vi "ConvertPB_Triggers.vi"(0 "PB VLIW Array in":T2(array[cluster]) {"Output Bits" format="%x"}, 1 "Definitions":T1={"External MemorySize"=32768, "Internal Memory Size"=512, "Overhead Ticks"=3, "Min Delay Loops"=3, "Loop Count Correction"=1, "Long Delay Loop Count Correction"=2, "Min Instruction Ticks"=6, "Long Delay Ticks"=4294967295, "Clock Period (s)"=1e-08, "Overhead Time (s)"=3e-08, "Min Instruction Cycle Time (s)"=9e-08, "Long Delay Time (s) "=42.94967298} {"Long Delay Time (s)" format="%.8p"; "Min Instruction Cycle Time (s)" format="%.0p"; "Overhead Time (s)" format="%.0p"; "Clock Period (s)" format="%.0p"; "Long Delay Ticks" format="%.0x"}, 2 "error in (no error)":errorcluster, 3 "Full trigger mask":u32 format="%x") -> (5 "PB VLIW Array out":T2(array[cluster]) {"Output Bits" format="%x"}, 6 "error out":errorcluster)   [LabVIEW 2013, in "PulseBlaster.lvlib"]
uses:
  PulseBlaster.lvlib
panel:
  in  "BeginLoop pointer":u32
  # "(Period*Long D Ticks)+Overhead time"
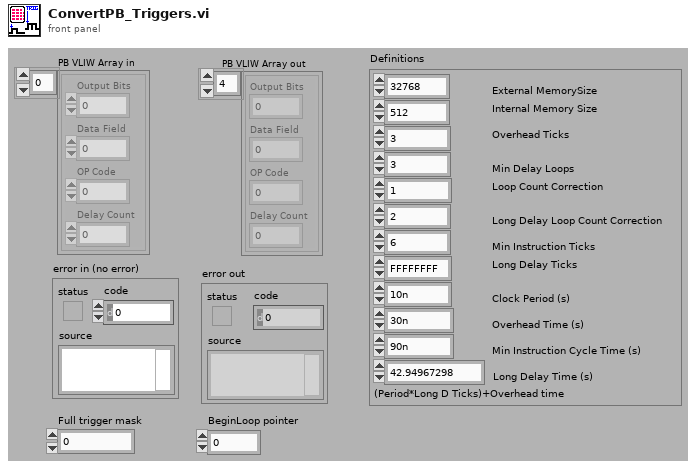
[diagram p1: front panel]
types:
  T1 = cluster{"External MemorySize":u16, "Internal Memory Size":u16, "Overhead Ticks":u8, "Min Delay Loops":u8, "Loop Count Correction":u8, "Long Delay Loop Count Correction":u8, "Min Instruction Ticks":u8, "Long Delay Ticks":u64, "Clock Period (s)":dbl, "Overhead Time (s)":dbl, "Min Instruction Cycle Time (s)":dbl, "Long Delay Time (s) ":dbl}
  T2 = cluster{"Output Bits":u32, "Data Field":u32, "OP Code":u8, "Delay Count":u64}[]
  T3 = cluster{"Output Bits":u32, "Data Field":u32, "OP Code":u8, "Delay Count":u64}
  T4 = cluster{"Output Bits":u32, "Data Field":u32, "OP Code":i32, "Delay Count":u64}[]
  T5 = cluster{"Output Bits":u32, "BeginLoop pointer":u32, "OP Code":u8, "Delay Count":u64}
  T6 = cluster{"Output Bits":u32, "BeginLoop pointer":u32, "OP Code":i32, "Delay Count":u64}[]
  T7 = cluster{"Output Bits":u32, "Data Field":u32, "OP Code":u8, u64}
  T8 = cluster{"Output Bits":u32, i32, i32, "Min Instruction Ticks":u8}
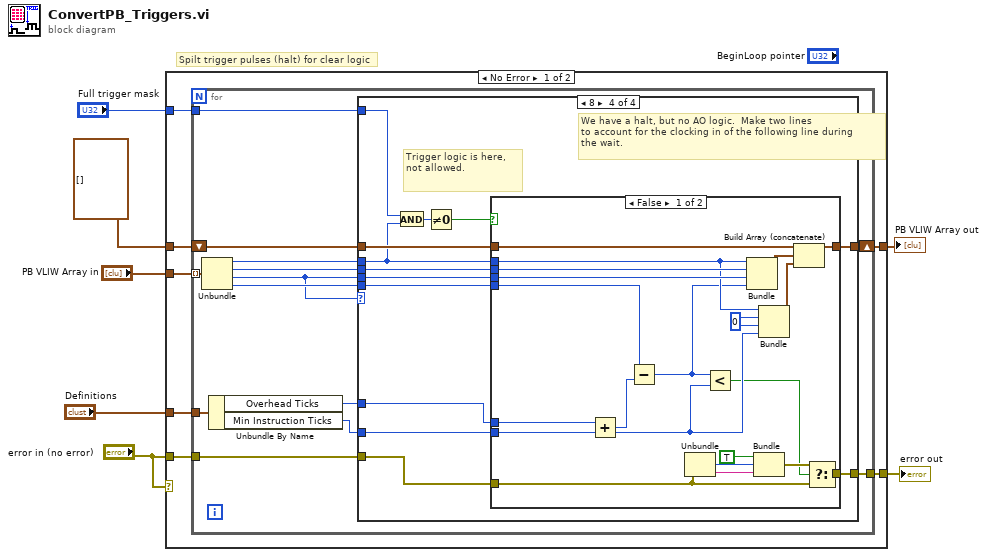
[diagram p0: block diagram]
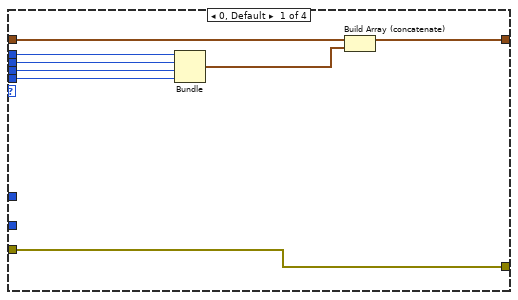
[diagram p2: hidden frame]
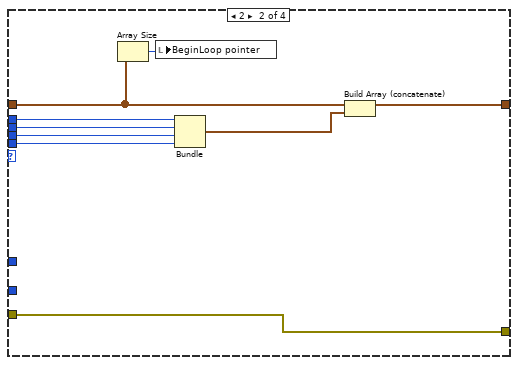
[diagram p3: hidden frame]
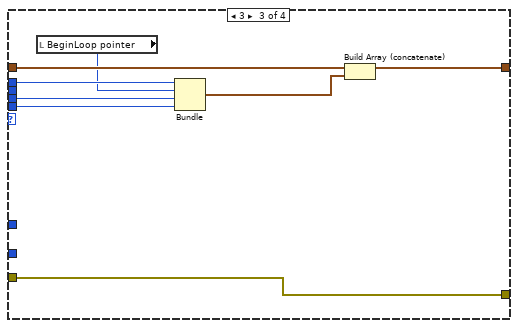
[diagram p4: hidden frame]
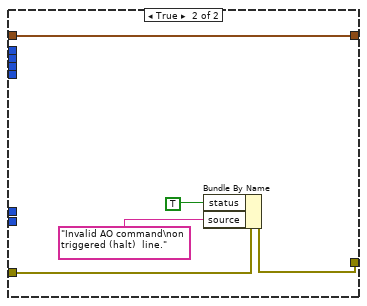
[diagram p5: hidden frame]
diagram:
  # "Spilt trigger pulses (halt) for clear logic"
  n1 = case shown="No Error" "error in (no error)" {
    tunnel: T2 [] -> [w14 _]
    tunnel: [w13 w92] -> w6
    tunnel: "PB VLIW Array in" -> [w12 w92]
    tunnel: "error in (no error)" -> [w11 w91]
    tunnel: [w10 w91] -> w4
    tunnel: "Full trigger mask" -> [w9 _]
    tunnel: "Definitions" -> [w8 _]
    frame No Error {
      n2 = for {
        tunnel: w12 -> [w27] mode=indexing
        shift-right: [w21] -> w13
        shift-left: w14 -> [w24]
        tunnel: w11 -> [w23]
        tunnel: [w22] -> w10
        tunnel: w9 -> [w18]
        tunnel: w8 -> [w17]
        n3 = Unbundle(w27) -> ("Output Bits"=w19:u32, "Data Field"=w26:u32, "OP Code"=w20:u8, "Delay Count"=w25:u64)
        n4 = Unbundle By Name(w17) -> ("Overhead Ticks"=w16:u8, "Min Instruction Ticks"=w15:u8)
        n5 = case shown="8" w20 {
          tunnel: w26 -> [w35 w44 _ w65]
          tunnel: w20 -> [w34 w43 w52 w64]
          tunnel: w25 -> [w33 w42 w51 w63]
          tunnel: w24 -> [w32 w36 w50 w62]
          tunnel: w23 -> [w31 w41 w49 w61]
          tunnel: [w31 w41 w49 w60] -> w22
          tunnel: w16 -> [_ _ _ w58]
          tunnel: w15 -> [_ _ _ w57]
          tunnel: w19 -> [w30 w40 w48 w56]
          tunnel: [w29 w39 w47 w59] -> w21
          tunnel: w18 -> [_ _ _ w53]
          frame 0, Default {
            n6 = Bundle("Output Bits"=w30, "Data Field"=w35, "OP Code"=w34, "Delay Count"=w33) -> (w28:T3)  [unwired: 1 out]
            n7 = Build Array (concatenate)(w32, w28) -> (w29:T4)
          }
          frame 2 {
            n8 = Array Size(array=w36) -> (size(s)=w37:i32)
            n9 = local write "BeginLoop pointer"(w37) -> ()
            n10 = Bundle("Output Bits"=w40, "Data Field"=w44, "OP Code"=w43, "Delay Count"=w42) -> (w38:T3)  [unwired: 1 out]
            n11 = Build Array (concatenate)(w36, w38) -> (w39:T4)
          }
          frame 3 {
            n12 = local read "BeginLoop pointer"() -> (w45:u32)
            n13 = Bundle("Output Bits"=w48, "BeginLoop pointer"=w45, "OP Code"=w52, "Delay Count"=w51) -> (w46:T5)  [unwired: 1 out]
            n14 = Build Array (concatenate)(w50, w46) -> (w47:T6)
          }
          frame 8 {
            # "Trigger logic is here,\nnot allowed."
            # "We have a halt, but no AO logic.  Make two lines\nto account for the clocking in of the following line during\nthe wait."
            n15 = And(x=w53, y=w56) -> (x .and. y?=w55:u32)
            n16 = Not Equal To 0?(x=w55) -> (x != 0?=w54:bool)
            n17 = case shown="False" w54 {
              tunnel: w65 -> [w85 _]
              tunnel: w64 -> [w84 _]
              tunnel: w63 -> [w67 _]
              tunnel: w62 -> [w83 w86]
              tunnel: w61 -> [w82 w90]
              tunnel: [w81 w89] -> w60
              tunnel: [w80 w86] -> w59
              tunnel: w58 -> [w79 _]
              tunnel: w57 -> [w78 _]
              tunnel: w56 -> [w68 _]
              frame False {
                w71 = 0
                n18 = Add(x=w79, y=w78) -> (x+y=w70:u8)
                n19 = Subtract(x=w67, y=w70) -> (x-y=w66:u64)
                n20 = Unbundle(w82) -> ("code"=w75:i32, "source"=w76:string)  [unwired: 1 out]
                n21 = Less?(x=w66, y=w78) -> (x < y?=w69:bool)
                n22 = Bundle("Output Bits"=w68, "Data Field"=w85, "OP Code"=w84, w66) -> (w73:T7)  [unwired: 1 out]
                n23 = Bundle(TRUE, "code"=w75, "source"=w76) -> (w74:cluster{bool, "code":i32, "source":string})  [unwired: 1 out]
                n24 = Bundle("Output Bits"=w68, w71, w71, "Min Instruction Ticks"=w78) -> (w72:T8)  [unwired: 1 out]
                n25 = Build Array (concatenate)(w83, w73, w72) -> (w80:T4)
                n26 = Select(t=w74, s=w69, f=w82) -> (s? t:f=w81:errorcluster)
              }
              frame True {
                n27 = Bundle By Name(cluster=w90, "status"=TRUE, "source"="Invalid AO command\non triggered (halt)  line.") -> (w89:errorcluster)
              }
            }
          }
        }
      }
    }
    frame Error {
    }
  }
  "error out" <- w4
  "PB VLIW Array out" <- w6
